vi "Add Child.vi"(8 "Error In":errorcluster, 10 "Child":refnum<class "Abstract.lvclass">, 11 "Non-Terminal In":refnum<class "NonTerminal.lvclass">) -> (0 "Error Out":errorcluster, 3 "Non-Terminal Out":refnum<class "NonTerminal.lvclass">)   [LabVIEW 2018, in "Toolkit.lvlib" / "Nodes.lvlib" / "NonTerminal.lvclass"]
uses:
  NonTerminal.lvclass
  Abstract/Abstract.lvclass
  NonTerminal.lvclass/NonTerminal.ctl
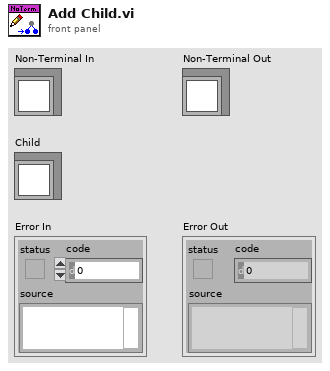
[diagram p1: front panel]
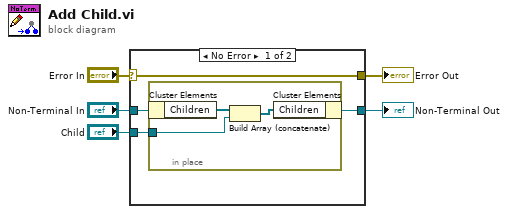
[diagram p0: block diagram]
diagram:
  n1 = case shown="No Error" "Error In" {
    selector: "Error In" -> [w9 w14]
    tunnel: [w9 w14] -> w4
    tunnel: [w6 w13] -> w2
    tunnel: "Non-Terminal In" -> [w8 w13]
    tunnel: "Child" -> [w7 _]
    frame No Error {
      n2 = in-place {
        in-place-border: w7 -> [w11]
        n3 = in-place-cluster #1(w8) -> ("Children"=w12:refnum<class "Abstract.lvclass">[])
        n4 = Build Array (concatenate)(w12, w11) -> (w10:refnum<class "Abstract.lvclass">[])
        n5 = in-place-cluster #1("Children"=w10) -> (w6:refnum<class "NonTerminal.lvclass">)
      }
    }
    frame Error {
    }
  }
  "Error Out" <- w4
  "Non-Terminal Out" <- w2
